vi "Prompt File Dialog.vi"(4 "pattern (all files)":string, 6 "pattern label":string, 7 "prompt":string, 8 "error in":errorcluster, 9 "Check if directory (T)":bool=TRUE, 10 "default name":string, 11 "File Path":path) -> (0 "error out":errorcluster, 3 "selected path":path)   [LabVIEW 2020]
doc: "If file path is empty (default) or is <Not A Path> or is a directory, the VI displays a dialog box from which you can select a file. Error 43 occurs if you cancel the dialog box."
uses:
  <vilib>/Utility/error.llb/Error Cluster From Error Code.vi
  <vilib>/ErrorRing/Error Ring.xnode
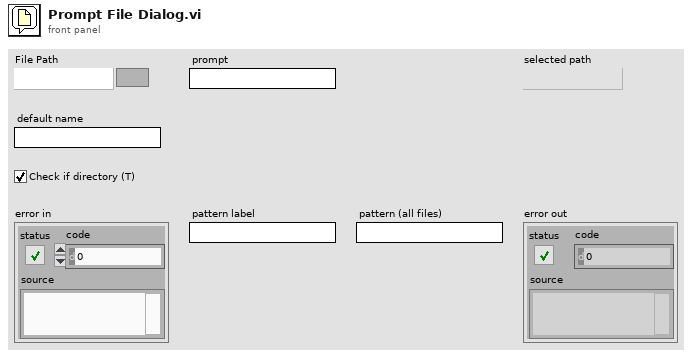
[diagram p1: front panel]
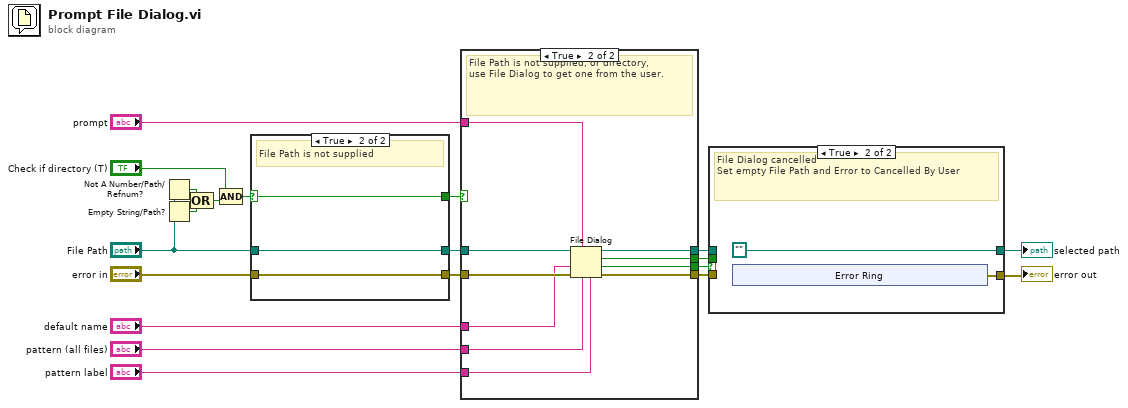
[diagram p0: block diagram]
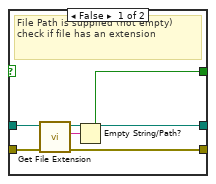
[diagram p2: hidden frame]
diagram:
  n1 = Not A Number/Path/Refnum?(number/path/refnum="File Path") -> (NaN/Path/Refnum?=w17:bool)
  n2 = Empty String/Path?(string/path="File Path") -> (empty?=w16:bool)
  n3 = Compound Arithmetic op=OR(w17, w16) -> (w9:bool)
  n4 = Compound Arithmetic op=AND("Check if directory (T)", w9) -> (w2:bool)
  n5 = case shown="True" w2 {
    selector: w2 -> [_ w27]
    tunnel: "File Path" -> [w26 w29]
    tunnel: "error in" -> [w25 w28]
    tunnel: [w23 w28] -> w5
    tunnel: [w24 w29] -> w4
    tunnel: [w21 w27] -> w3
    frame False {
      # "File Path is supplied (not empty) \ncheck if file has an extension"
      n6 = call <vilib>:"Get File Extension.vi"("error in (no error)"=w25, "file"=w26) -> ("error out"=w23:errorcluster, "lowercase file extension"=w22:string, "dup file"=w24:path)  [unwired: 5 in, 2 out]
      n7 = Empty String/Path?(string/path=w22) -> (empty?=w21:bool)
    }
    frame True {
      # "File Path is not supplied"
    }
  }
  n8 = case shown="True" w3 {
    tunnel: w5 -> [w30 w41]
    tunnel: [w30 w40] -> w13
    tunnel: "pattern (all files)" -> [_ w39]
    tunnel: "pattern label" -> [_ w38]
    tunnel: "default name" -> [_ w37]
    tunnel: [w31 w36] -> w14
    tunnel: w4 -> [w31 w35]
    tunnel: "prompt" -> [_ w34]
    tunnel: [_ w33] -> w10
    tunnel: [_ w32] -> w15
    frame False {
      # "File Path is supplied (not empty and not a directory)"
    }
    frame True {
      # "File Path is not supplied, or directory,\nuse File Dialog to get one from the user."
      n9 = File Dialog(4:w38, 6:w39, 7:w34, 8:w41, 9:w37, 11:w35) -> (0:w40:errorcluster, 1:w32:bool, 2:w33:bool, 3:w36:path)  [unwired: 1 in]
    }
  }
  n10 = case shown="True" w15 {
    tunnel: w14 -> [w43 _]
    tunnel: w13 -> [w42 _]
    tunnel: [w43 path ""] -> w12
    tunnel: [w42 w44] -> w11
    tunnel: w10 -> [_ _]
    frame False {
      # "File path supplied or selected"
    }
    frame True {
      # "File Dialog cancelled\nSet empty File Path and Error to Cancelled By User"
      n11 = xnode "Error Ring"() -> ("error out"=w44:errorcluster)
    }
  }
  "error out" <- w11
  "selected path" <- w12
